vi "SetupPump.vi"(8 "error in (no error)":errorcluster, 9 "Set rate":dbl format="%#_4g", 10 "dia (mm)":dbl=0.1 caption="Dia (mm)" min=0.1 max=50.0, 11 "VISA Refnum in":refnum<visa-resource-name>) -> (0 "error out":errorcluster, 2 "rate":dbl, 3 "VISA Refnum out":refnum<visa-resource-name>)   [LabVIEW 2020]
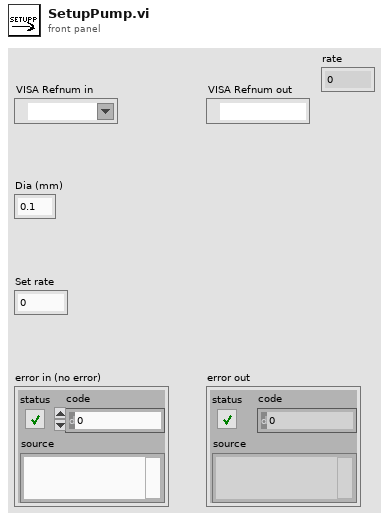
[diagram p1: front panel]
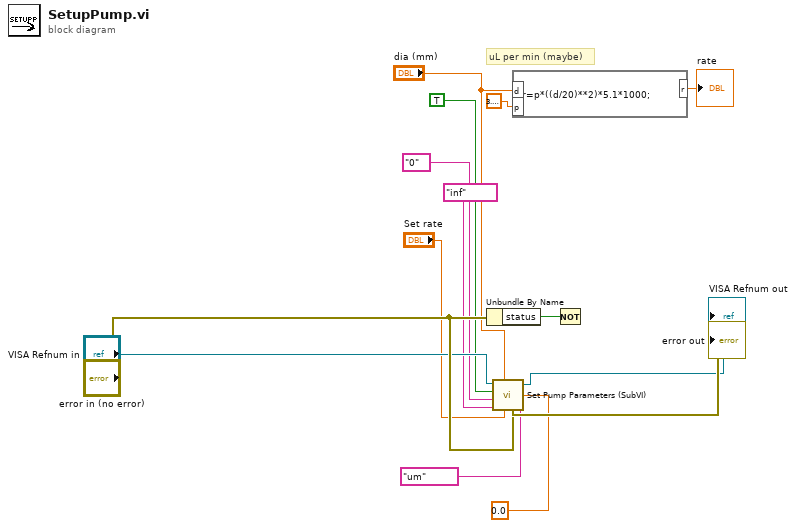
[diagram p0: block diagram]
diagram:
  # "uL per min (maybe)"
  n1 = Unbundle By Name("error in (no error)") -> ("status"=w2:bool)
  n2 = call "Set Pump Parameters (SubVI).vi"("Units"="um", "error in"="error in (no error)", "Target Volume"=0.0 ("Target Vol"), "Flow rate"="Set rate", "Direction"="inf", "Pump Add"="0" ("Address"), "diameter (mm)"="dia (mm)", "Send"=TRUE, "VISA resource name in"="VISA Refnum in") -> ("VISA resource name out"=→"VISA Refnum out":refnum<visa-resource-name>, "error out"=→"error out":errorcluster)
  n3 = formula code="r=p*((d/20)**2)*5.1*1000;"("d"="dia (mm)", "p"=3.141592653589793) -> ("r"=→"rate":dbl)
  n4 = Not(x=w2) -> ()  [unwired: 1 out]
